vi "Run Game.vi"() -> ()   [LabVIEW 2024]
uses:
  Controller/Car Control.vi
  FormulaG/FormulaG App/FormulaG App.lvclass
  Controller/Controller.lvlib
panel:
  in  "Port":u16=10027
  in  "Run External":bool
  # "Run this VI to play!"
  # "Use Run External if you're running inside of a VM and need to run the graphics in a browser on the host sysyem for performance."
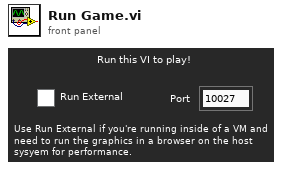
[diagram p1: front panel]
types:
  T1 = enum32{"Invalid", "Standard", "Closed", "Hidden", "Minimized", "Maximized"}
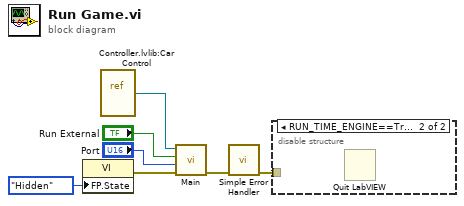
[diagram p0: block diagram]
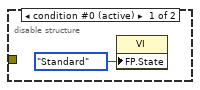
[diagram p2: hidden frame]
diagram:
  n1 = property class="VI"("FP.State"=T1."Hidden" ("Front Panel Window:State")) -> (error out=w5:errorcluster)  [unwired: 2 in, 1 out]
  n2 = vi-ref "Controller.lvlib:Car Control.vi"() -> (w7:refnum<vi>)
  n3 = call "Main.vi"("error in (no error)"=w5, "Port"="Port", "Run External"="Run External", "Control VI"=w7) -> ("error out"=w4:errorcluster)  [unwired: 7 in]
  n4 = call <vilib>:"Simple Error Handler.vi"("error in (no error)"=w4) -> ("error out"=w3:errorcluster)  [unwired: 4 in, 4 out]
  n5 = disable-structure shown="RUN_TIME_ENGINE==True" {
    disable-tunnel: w3 -> [_ _]
    frame condition #0 (active) {
      n6 = property class="VI"("FP.State"=T1."Standard" ("Front Panel Window:State")) -> ()  [unwired: 2 in, 2 out]
    }
    frame condition #1 {
      n7 = Quit LabVIEW() -> ()  [unwired: 1 in]
    }
  }
